vi "Main RT.vi"() -> ()   [LabVIEW 2015]
uses:
  <vilib>/RioEmbeddedCAN/RioEmbeddedCAN.llb/CANFrameControl.ctl
  <vilib>/Platform/TimedLoop/XDataNode/timing_clust.ctl
  <vilib>/Platform/TimedLoop/XDataNode/nitl_modes.ctl
  <vilib>/Platform/TimedLoop/XDataNode/wakeup.ctl
  <vilib>/FPGAPlugInAG/sbRIO-9636/niLvFpga_Open_sbRIO-9636.vi
  <vilib>/rvi/interface/common/dynamic/niFpgaDynamicAddResources.vi
  <vilib>/FPGAPlugInAG/Dynamic/niLvFpga_Reset_Dynamic.vi
  <vilib>/FPGAPlugInAG/Dynamic/niLvFpga_Run_Dynamic.vi
  <vilib>/FPGAPlugInAG/Dynamic/niLvFpga_Close_Dynamic.vi
  <vilib>/Platform/TimedLoop/XDataNode/XDataNode.xnode
  <vilib>/rvi/interface/nirviOpenFPGA/nirviOpenFPGA.xnode
  FPGA Bitfiles/Raptorv2_FPGATarget_FPGAMain_SQ-6zSZl0hY.lvbitx
  FPGA/Main FPGA.vi
  <vilib>/rvi/interface/nirviMethod/nirviMethod.xnode
  <vilib>/rvi/interface/nirviCloseFPGA/nirviCloseFPGA.xnode
  <vilib>/Platform/TimedLoop/XDataNode/XDNodeRunTimeDep.lvlib
  <vilib>/Instr/_visa.llb/VISA Configure Serial Port (Instr).vi
panel:
  out "longitude (deg) 2":dbl format="%#_8g"
  out "latitude (deg) 2":dbl format="%#_8g"
  in  "VISA resource name":refnum<visa-resource-name>="ASRL1::INSTR"
  out "longitude (deg)":i64
  out "latitude (deg)":i64
  out "GPS data":T1 {"oldest read timestamp" format="%^<%.3X\n%x>T"; "latitude (deg)" format="%#_10g"; "longitude (deg)" format="%#_10g"}
  out "Numeric 2":i32
  out "Numeric":i32
  out "okres 1000":dbl
  out "wyczyszczona":bool=TRUE
  in  "Wyczyśćkolejke":bool
  in  "stop wysylanie":bool
  out "odczytany CAN":T2 {"type" items=["CAN Data", "CAN Remote"]; "identifier" format="%.0x"}
  out "ile nowych mesagy":dbl
  in  "odczyt":bool=TRUE
  out "okres 100":dbl
  out "ilosc mesagy":dbl
  in  "ramki 2":bool
  out "Frames":string[][](table)
  in  "stop odczyt can":bool
  in  "Hexadecimal?":bool
  in  "stop zapis can":bool
  out "new data":bool
  out "ramki jazdy":T2[](array[typedef]) {"type" items=["CAN Data", "CAN Remote"]; "identifier" format="%.0x"}
  in  "odbior udp":bool
  out "ramki konf":T2 {"type" items=["CAN Data", "CAN Remote"]; "identifier" format="%.0x"}
  in  "Number of Frames to Display":i32=5
  in  "receive queue size":u32=500
  in  "baud rate":u32=500000
  in  "interface index":u32
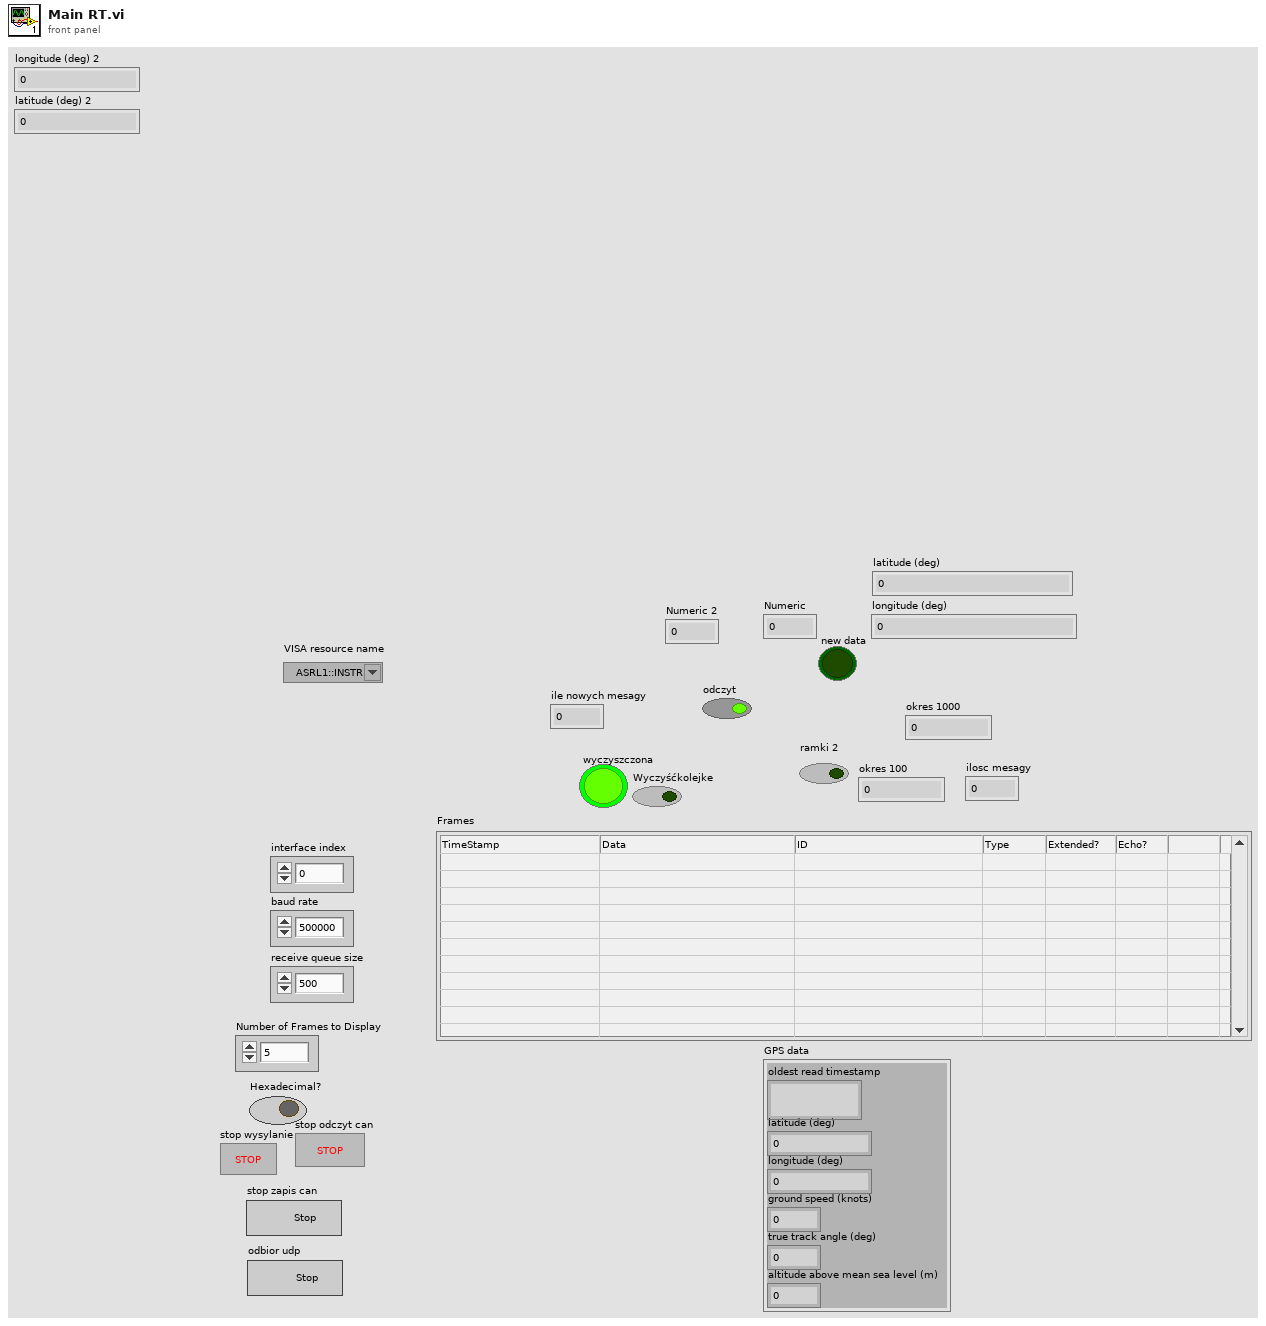
[diagram p1: front panel]
types:
  T1 = cluster{"oldest read timestamp":timestamp, "latitude (deg)":dbl, "longitude (deg)":dbl, "ground speed (knots)":dbl, "true track angle (deg)":dbl, "altitude above mean sea level (m)":dbl}
  T2 = typedef "CANFrameControl.ctl" = cluster{"identifier":u32, "extended?":bool, "type":u8, "payload":u8[]}
  T3 = typedef "XDNodeRunTimeDep.lvlib/timing_clust.ctl" = cluster{"Expected End [f-1]":u64, "Actual End [f-1]":u64, "Finished Late? [f-1]":bool, "Expected End [i-1]":u64, "Actual End [i-1]":u64, "Finished Late? [i-1]":bool, "Expected Start [i]":u64, "Actual Start [i]":u64, "Expected Start [f]":u64, "Actual Start [f]":u64, "Source Name":string, "Structure Name":string, "Period":i64, "Deadline":i64, "Offset":i64, "Start":i64, "Priority":i32, "Timeout":i32, "Mode":T4, "Wakeup Reason":T5, "Error":errorcluster, "Source Type":string, "Secondary Source Type":string, "Global End Time":u64, "Global Start Time":u64, "Frame Duration":u64, "Iteration Duration":u64, "Assigned CPU":i32, "I/O Scan Engine Mode":u32}
  T4 = typedef "XDNodeRunTimeDep.lvlib/nitl_modes.ctl" = enum32{"No Change", "Process missed periods, maintain original phase", "Discard missed periods, maintain original phase", "Process missed periods, ignore original phase", "Discard missed periods, ignore original phase"}
  T5 = typedef "XDNodeRunTimeDep.lvlib/wakeup.ctl" = enum32{"Normal", "Aborted", "Asynchronous wakeup", "Timing source error", "Timed loop error", "Timeout"}
  T6 = cluster{"latitude (deg)":i64, "longitude (deg)":i64}
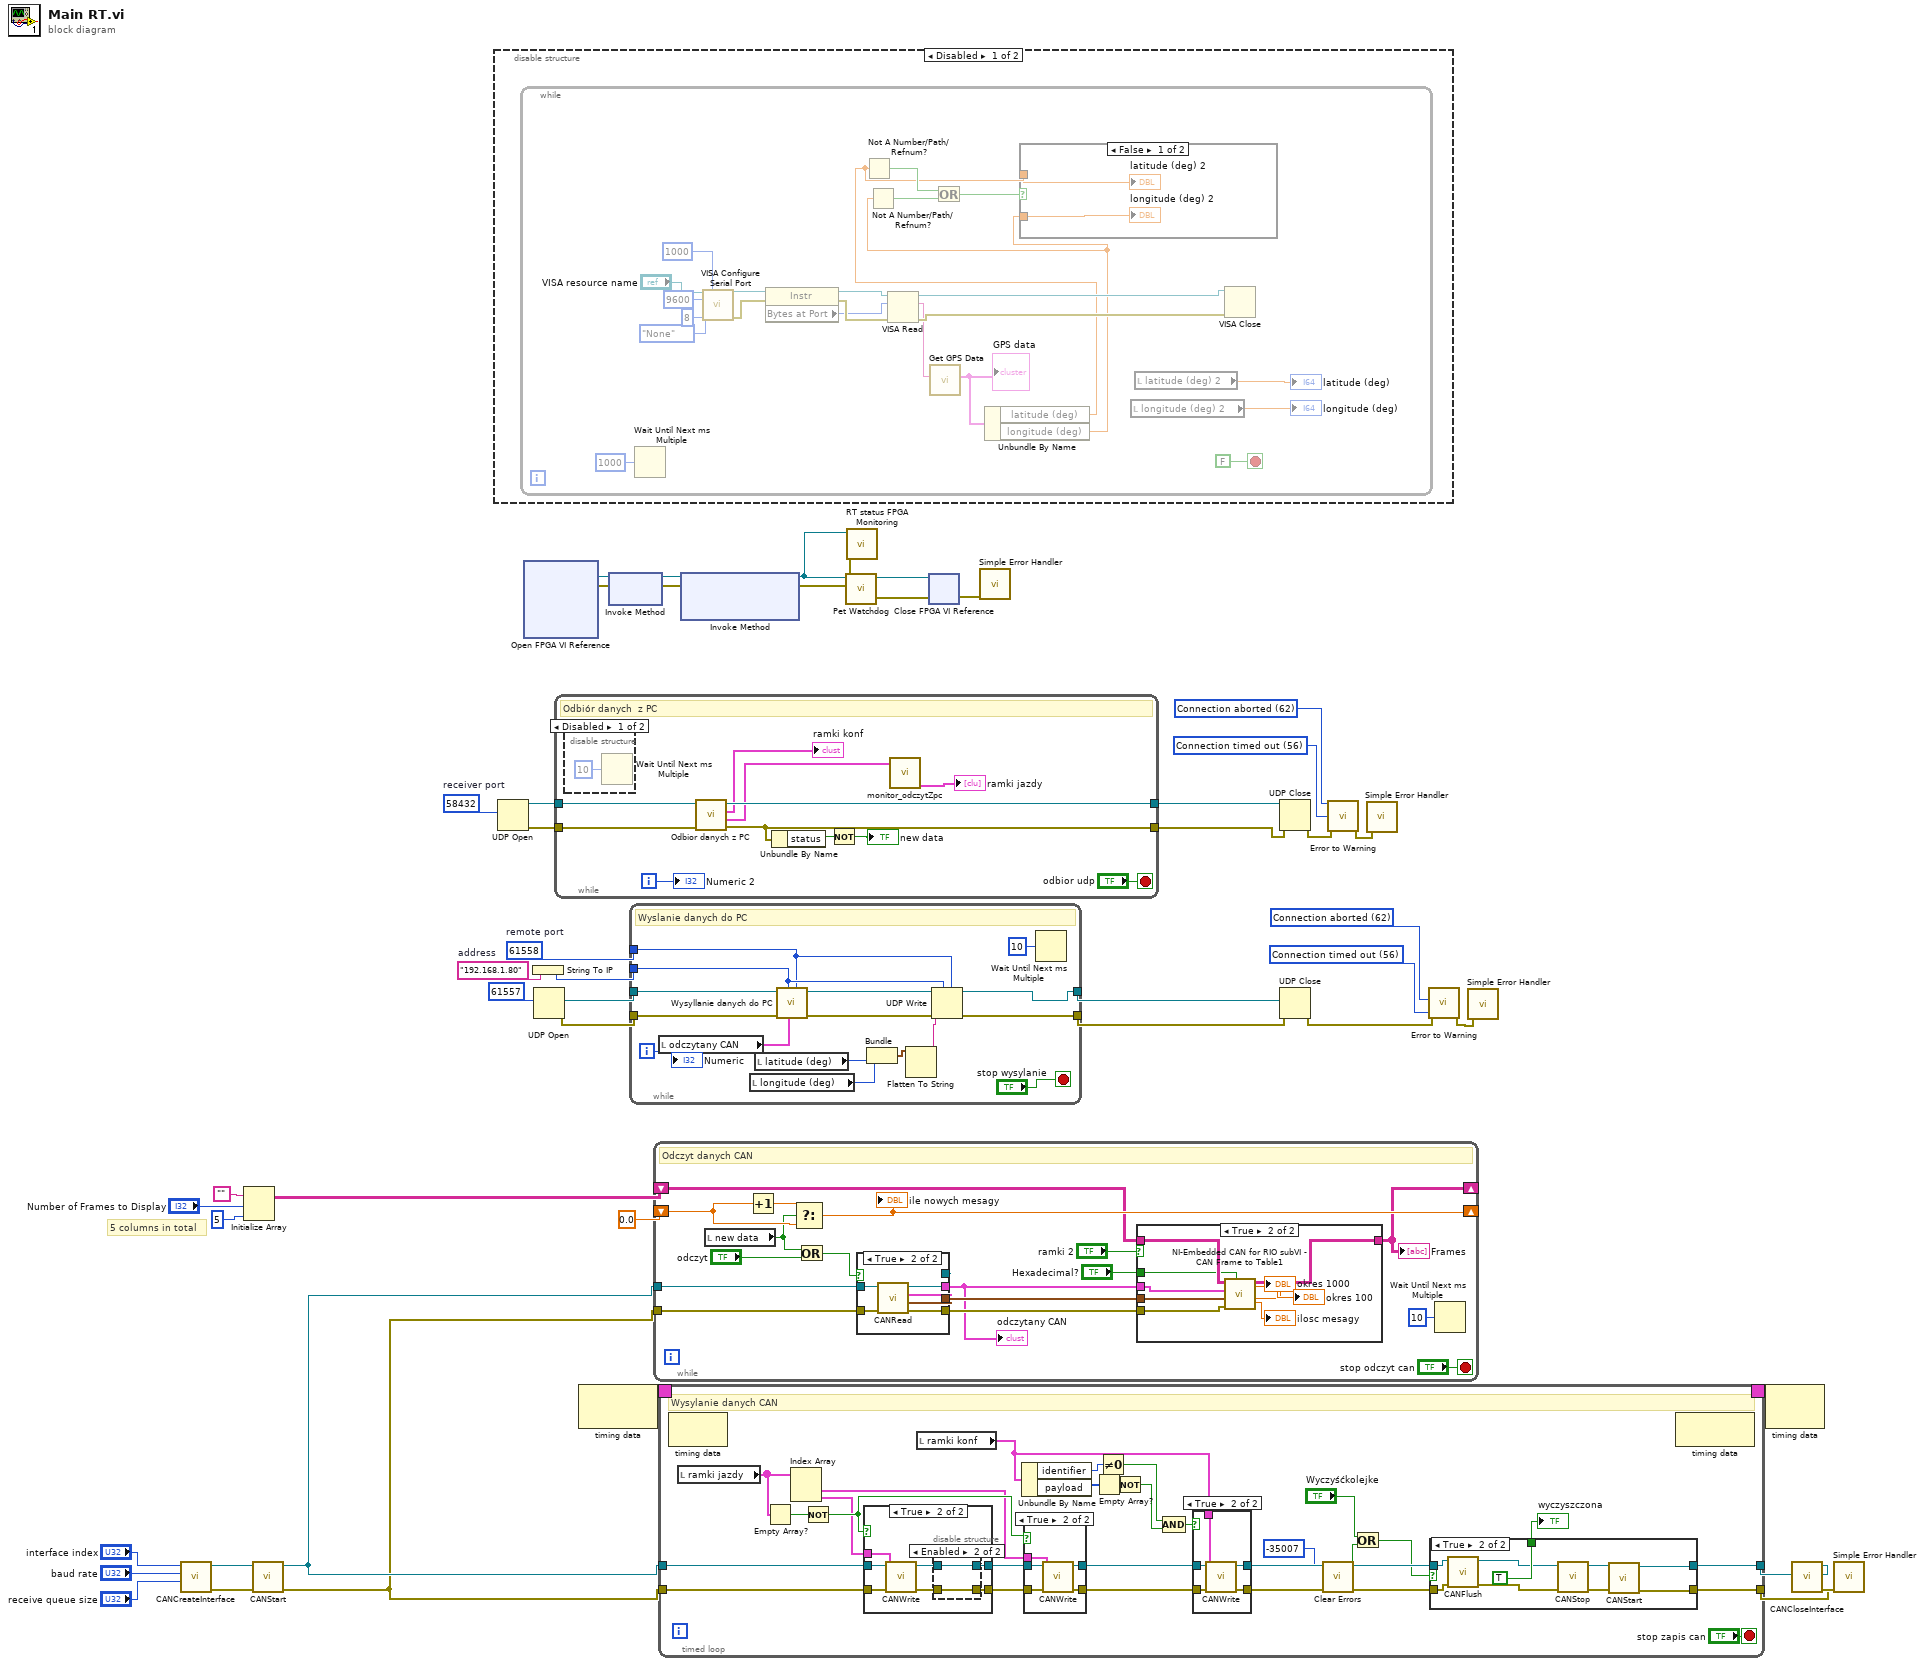
[diagram p0: block diagram]
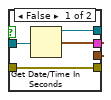
[diagram p6: hidden frame]
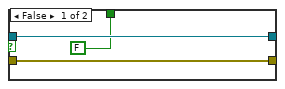
[diagram p7: hidden frame]
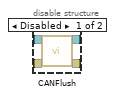
[diagram p11: hidden frame]
diagram:
  w2 = u16 58432  # receiver port
  w6 = 56 items=["No Error", "Argument Error", "Memory Full", "Out of Zone", "End of File", "File Already Open", "Generic File IO Error", "File Not Found", "File Permission Error", "Disk Full", "Duplicate Path", "Too Many Files Open", "Not Enabled", "Resource File Not Found", "Cannot Add Resource", "Resource Not Found", "Image Not Found", "Image Memory Error", "Pen Does Not Exist", "Config Bad Type", "Config Token Not Found", "Config Parse Error", "Config Memory Error", "Bad External Code Format", "Bad External Code Offset", "External Code Not Present", "Null Window", "Destroy Window Mixup", "Null Menu", "Print Aborted", "Bad Print Record", "Print Driver Error", "Windows Error During Print", "Memory Error During Print", "Print Dialog Error", "Generic Print Error", "Invalid Device Refnum", "Device Not Found", "Device Parameter Error", "Device Unit Error", "Can't Open Device", "Device Call Aborted", "Generic Error", "Cancelled By User", "Object ID Too Low", "Object ID Too High", "Object Not In Heap", "Unknown Heap", "Bad DefProc ID", "DefProc Not In Table", "Message Out Of Range", "Null Method", "Unknown Message", "Manager Call Not Supported", "Bad address", "Connection In progress", "Connection timed out", "Connection is already in progress", "Network attribute not supported", "Network error", "Address in use", "System out of memory", "Connection aborted", "Connection refused", "Connection is not connected", "Connection is already connected", "Connection closed", "Initialize error (interapplication manager)", "Bad occurrence", "Wait on unbound occurrence handler", "Occurrence queue overflow", "Bad path", "Semaphore not signaled", "Unrecognized type (interapplication manager)"] ("3rd Error to Convert")
  w5 = 62 items=["No Error", "Argument Error", "Memory Full", "Out of Zone", "End of File", "File Already Open", "Generic File IO Error", "File Not Found", "File Permission Error", "Disk Full", "Duplicate Path", "Too Many Files Open", "Not Enabled", "Resource File Not Found", "Cannot Add Resource", "Resource Not Found", "Image Not Found", "Image Memory Error", "Pen Does Not Exist", "Config Bad Type", "Config Token Not Found", "Config Parse Error", "Config Memory Error", "Bad External Code Format", "Bad External Code Offset", "External Code Not Present", "Null Window", "Destroy Window Mixup", "Null Menu", "Print Aborted", "Bad Print Record", "Print Driver Error", "Windows Error During Print", "Memory Error During Print", "Print Dialog Error", "Generic Print Error", "Invalid Device Refnum", "Device Not Found", "Device Parameter Error", "Device Unit Error", "Can't Open Device", "Device Call Aborted", "Generic Error", "Cancelled By User", "Object ID Too Low", "Object ID Too High", "Object Not In Heap", "Unknown Heap", "Bad DefProc ID", "DefProc Not In Table", "Message Out Of Range", "Null Method", "Unknown Message", "Manager Call Not Supported", "Bad address", "Connection In progress", "Connection timed out", "Connection is already in progress", "Network attribute not supported", "Network error", "Address in use", "System out of memory", "Connection aborted", "Connection refused", "Connection is not connected", "Connection is already connected", "Connection closed", "Initialize error (interapplication manager)", "Bad occurrence", "Wait on unbound occurrence handler", "Occurrence queue overflow", "Bad path", "Semaphore not signaled", "Unrecognized type (interapplication manager)"] ("1st Error to Convert")
  w13 = u16 61558  # remote port
  w14 = "192.168.1.80"  # address
  w17 = 56 items=["No Error", "Argument Error", "Memory Full", "Out of Zone", "End of File", "File Already Open", "Generic File IO Error", "File Not Found", "File Permission Error", "Disk Full", "Duplicate Path", "Too Many Files Open", "Not Enabled", "Resource File Not Found", "Cannot Add Resource", "Resource Not Found", "Image Not Found", "Image Memory Error", "Pen Does Not Exist", "Config Bad Type", "Config Token Not Found", "Config Parse Error", "Config Memory Error", "Bad External Code Format", "Bad External Code Offset", "External Code Not Present", "Null Window", "Destroy Window Mixup", "Null Menu", "Print Aborted", "Bad Print Record", "Print Driver Error", "Windows Error During Print", "Memory Error During Print", "Print Dialog Error", "Generic Print Error", "Invalid Device Refnum", "Device Not Found", "Device Parameter Error", "Device Unit Error", "Can't Open Device", "Device Call Aborted", "Generic Error", "Cancelled By User", "Object ID Too Low", "Object ID Too High", "Object Not In Heap", "Unknown Heap", "Bad DefProc ID", "DefProc Not In Table", "Message Out Of Range", "Null Method", "Unknown Message", "Manager Call Not Supported", "Bad address", "Connection In progress", "Connection timed out", "Connection is already in progress", "Network attribute not supported", "Network error", "Address in use", "System out of memory", "Connection aborted", "Connection refused", "Connection is not connected", "Connection is already connected", "Connection closed", "Initialize error (interapplication manager)", "Bad occurrence", "Wait on unbound occurrence handler", "Occurrence queue overflow", "Bad path", "Semaphore not signaled", "Unrecognized type (interapplication manager)"] ("3rd Error to Convert")
  w18 = 62 items=["No Error", "Argument Error", "Memory Full", "Out of Zone", "End of File", "File Already Open", "Generic File IO Error", "File Not Found", "File Permission Error", "Disk Full", "Duplicate Path", "Too Many Files Open", "Not Enabled", "Resource File Not Found", "Cannot Add Resource", "Resource Not Found", "Image Not Found", "Image Memory Error", "Pen Does Not Exist", "Config Bad Type", "Config Token Not Found", "Config Parse Error", "Config Memory Error", "Bad External Code Format", "Bad External Code Offset", "External Code Not Present", "Null Window", "Destroy Window Mixup", "Null Menu", "Print Aborted", "Bad Print Record", "Print Driver Error", "Windows Error During Print", "Memory Error During Print", "Print Dialog Error", "Generic Print Error", "Invalid Device Refnum", "Device Not Found", "Device Parameter Error", "Device Unit Error", "Can't Open Device", "Device Call Aborted", "Generic Error", "Cancelled By User", "Object ID Too Low", "Object ID Too High", "Object Not In Heap", "Unknown Heap", "Bad DefProc ID", "DefProc Not In Table", "Message Out Of Range", "Null Method", "Unknown Message", "Manager Call Not Supported", "Bad address", "Connection In progress", "Connection timed out", "Connection is already in progress", "Network attribute not supported", "Network error", "Address in use", "System out of memory", "Connection aborted", "Connection refused", "Connection is not connected", "Connection is already connected", "Connection closed", "Initialize error (interapplication manager)", "Bad occurrence", "Wait on unbound occurrence handler", "Occurrence queue overflow", "Bad path", "Semaphore not signaled", "Unrecognized type (interapplication manager)"] ("1st Error to Convert")
  # "5 columns in total"
  n1 = call <vilib>:"CANCreateInterface.vi"("receive queue size (5)"="receive queue size", "baud rate (125000 bps)"="baud rate", "interface index"="interface index") -> ("error out"=w45:errorcluster, "interface object out"=w35:refnum<k20>)  [unwired: 7 in]
  n2 = Initialize Array("" ("Empty String Constant"), "Number of Frames to Display", 5 ("dimension size")) -> (w34:string[][])
  n3 = call <vilib>:"CANStart.vi"("error in (no error)"=w45, "interface object in"=w35) -> ("error out"=w32:errorcluster, "interface object out"=w33:refnum<k20>)  [unwired: 8 in]
  n4 = disable-structure shown="Disabled" {
    frame Disabled {
      n5 = while {
        stop <- FALSE stop-if-true
        n6 = Wait Until Next ms Multiple(millisecond multiple=u32 1000) -> ()  [unwired: 1 out]
        n7 = call-poly "VISA Configure Serial Port"("VISA resource name"="VISA resource name", "timeout (10sec)"=u32 1000, "baud rate (9600)"=u32 9600, "data bits (8)"=u16 8, "parity (0:none)"=enum16{"None", "Odd", "Even", "Mark", "Space"}."None") -> ("VISA resource name out"=w67:refnum<visa-resource-name>, "error out"=w66:errorcluster)  [unwired: 9 in]
        n8 = property class="Instr"(reference=w67, error in=w66) -> (reference out=w68:refnum<visa-resource-name>, error out=w65:errorcluster, "Bytes at Port"=w61:u32)
        n9 = VISA Read(VISA resource name=w68, byte count=w61, error in (no error)=w65) -> (VISA resource name out=w69:refnum<visa-resource-name>, read buffer=w63:string, error out=w64:errorcluster)  [unwired: 1 out]
        n10 = call <vilib>:"Get GPS Data.vi"("sensor data"=w63) -> ("GPS data"=w62:T1)  [unwired: 8 in, 2 out]
        "GPS data" <- w62
        n11 = Unbundle By Name(w62) -> ("latitude (deg)"=w51:dbl, "longitude (deg)"=w49:dbl)
        n12 = Not A Number/Path/Refnum?(number/path/refnum=w51) -> (NaN/Path/Refnum?=w54:bool)
        n13 = Not A Number/Path/Refnum?(number/path/refnum=w49) -> (NaN/Path/Refnum?=w53:bool)
        n14 = Or(x=w54, y=w53) -> (x .or. y?=w52:bool)
        n15 = case shown="False" w52 {
          tunnel: w49 -> [w72 _]
          tunnel: w51 -> [w71 _]
          frame False {
            "longitude (deg) 2" <- w72
            "latitude (deg) 2" <- w71
          }
          frame True {
          }
        }
        n16 = local read "longitude (deg) 2"() -> (→"longitude (deg)":dbl)
        n17 = local read "latitude (deg) 2"() -> (→"latitude (deg)":dbl)
        n18 = VISA Close(VISA resource name=w69, error in (no error)=w64) -> ()  [unwired: 1 out]
      }
    }
    frame Enabled {
    }
  }
  n19 = UDP Open(11:w2) -> (port=w20:refnum<k16>, 0:w21:errorcluster)  [unwired: 4 in, 1 out]
  n20 = xnode "Open FPGA VI Reference"() -> ("FPGA VI Reference Out"=w26:refnum<k20>, "error out"=w27:errorcluster)  [unwired: 2 in]
  n21 = String To IP(1:w14) -> (0:w12:u32)
  n22 = UDP Open(11:u16 61557 ("port")) -> (port=w11:refnum<k16>, 0:w10:errorcluster)  [unwired: 4 in, 1 out]
  n23 = while {
    tunnel: w20 -> [w80]
    tunnel: w21 -> [w79]
    tunnel: [w82] -> w22
    tunnel: [w83] -> w3
    i -> [w78]
    stop <- "odbior udp" stop-if-true
    # "Odbiór danych  z PC"
    n24 = disable-structure shown="Disabled" {
      frame Disabled {
        n25 = Wait Until Next ms Multiple(millisecond multiple=u32 10) -> ()  [unwired: 1 out]
      }
      frame Enabled {
      }
    }
    n26 = call "Odbior danych z PC .vi"("error in (no error)"=w79, "connection ID"=w80) -> ("error out"=w82:errorcluster, "jazda"=w75:T2[], "konf"=→"ramki konf":T2, "connection ID out"=w83:refnum<k16>)  [unwired: 6 in]
    n27 = Unbundle By Name(w82) -> ("status"=w77:bool)
    n28 = Not(x=w77) -> (.not. x?=→"new data":bool)
    n29 = call "monitor_odczytZpc.vi"("ramki jazdy 2"=w75) -> ("ramki jazdy out"=→"ramki jazdy":T2[])  [unwired: 9 in, 1 out]
    "Numeric 2" <- w78
  }
  n30 = node-c288() -> (w47:T3)  [unwired: 1 in]
  n31 = xnode "Invoke Method"("FPGA VI Reference In"=w26, "error in"=w27) -> ("FPGA VI Reference Out"=w28:refnum<k20>, "error out"=w29:errorcluster)
  n32 = while {
    tunnel: w13 -> [w87]
    tunnel: w12 -> [w88]
    tunnel: w11 -> [w100]
    tunnel: w10 -> [w99]
    tunnel: [w86] -> w9
    tunnel: [w85] -> w8
    i -> [w95]
    stop <- "stop wysylanie" stop-if-true
    # "Wyslanie danych do PC"
    n33 = local read "odczytany CAN"() -> (w96:T2)
    n34 = local read "longitude (deg)"() -> (w89:i64)
    n35 = local read "latitude (deg)"() -> (w90:i64)
    n36 = call "Wysyllanie danych do PC .vi"("remote port"=w87, "odczytany CAN"=w96, "Numeric"=w88, "error in (no error)"=w99, "UDP Network Connection in"=w100) -> ("error out"=w94:errorcluster, "UDP Network Connection out"=w93:refnum<k16>)  [unwired: 5 in]
    n37 = Bundle("latitude (deg)"=w90, "longitude (deg)"=w89) -> (w91:T6)  [unwired: 1 in]
    n38 = Flatten To String(anything=w91) -> (data string=w92:string)  [unwired: 3 in, 2 out]
    n39 = UDP Write(address=w88, port or service name=w87, connection ID=w93, data in=w92, 8:w94) -> (error out=w85:errorcluster, 3:w86:refnum<k16>)  [unwired: 1 in]
    n40 = Wait Until Next ms Multiple(millisecond multiple=u32 10) -> ()  [unwired: 1 out]
    "Numeric" <- w95
  }
  n41 = while {
    shift-right: [w109] -> _
    shift-left: w34 -> [w108]
    shift-right: [w113] -> _
    shift-left: 0.0 -> [w114]
    tunnel: w33 -> [w117]
    tunnel: w32 -> [w116]
    stop <- "stop odczyt can" stop-if-true
    # "Odczyt danych CAN"
    n42 = local read "new data"() -> (w111:bool)
    n43 = Increment(x=w114) -> (x+1=w115:dbl)
    n44 = Select(t=w115, s=w111, f=w114) -> (s? t:f=w113:dbl)
    "ile nowych mesagy" <- w113
    n45 = Or(x=w111, y="odczyt") -> (x .or. y?=w110:bool)
    n46 = case shown="True" w110 {
      tunnel: w117 -> [w129 w136]
      tunnel: w116 -> [w130 w135]
      tunnel: [w128 w134] -> w107
      tunnel: [w130 w133] -> w106
      tunnel: [_ w131] -> w101
      tunnel: [w129 w132] -> _
      frame False {
        n47 = Get Date/Time In Seconds() -> (seconds since 1Jan1904=w128:timestamp)
      }
      frame True {
        n48 = call <vilib>:"CANRead.vi"("error in (no error)"=w135, "interface object in"=w136) -> ("error out"=w133:errorcluster, "timestamp"=w134:timestamp, "CAN frame"=w131:T2, "interface object out"=w132:refnum<k20>)  [unwired: 6 in]
      }
    }
    "odczytany CAN" <- w101
    n49 = case shown="True" "ramki 2" {
      tunnel: [w118 w127] -> w109
      tunnel: w108 -> [w118 w124]
      tunnel: w107 -> [_ w123]
      tunnel: w101 -> [_ w122]
      tunnel: w106 -> [_ w121]
      tunnel: "Hexadecimal?" -> [_ w120]
      frame False {
      }
      frame True {
        n50 = call "NI-Embedded CAN for RIO subVI - CAN Frame to Table1.vi"("Hexadecimal?"=w120, "error in (no error)"=w121, "timestamp"=w123, "CAN frame"=w122, "Input Array"=w124) -> ("okres 1000"=→"okres 1000":dbl, "Output Array"=w127:string[][], "ilosc mesagy"=→"ilosc mesagy":dbl, "okres 100"=→"okres 100":dbl)  [unwired: 2 in, 1 out]
      }
    }
    "Frames" <- w109
    n51 = Wait Until Next ms Multiple(millisecond multiple=u32 10) -> ()  [unwired: 1 out]
  }
  n52 = timed-loop "Timed Loop" {
    tunnel: w33 -> [w148]
    tunnel: w32 -> [w147]
    tunnel: [w146] -> w37
    tunnel: [w145] -> w36
    timing: w47 -> [_]
    timing-out: [_] -> w46
    stop <- "stop zapis can" stop-if-true
    # "Wysylanie danych CAN"
    n53 = node-c288() -> ()  [unwired: 1 in, 1 out]
    n54 = local read "ramki jazdy"() -> (w163:T2[])
    n55 = Empty Array?(array=w163) -> (empty?=w162:bool)
    n56 = Index Array(array=w163) -> (element #1=w160:T2, element #2=w159:T2)  [unwired: 2 in]
    n57 = Not(x=w162) -> (.not. x?=w161:bool)
    n58 = case shown="True" w161 {
      tunnel: w148 -> [w194 w202]
      tunnel: w147 -> [w195 w201]
      tunnel: [w194 w196] -> w164
      tunnel: [w195 w197] -> w165
      tunnel: w159 -> [_ w200]
      frame False {
      }
      frame True {
        n59 = call <vilib>:"CANWrite.vi"("error in (no error)"=w201, "CAN frame"=w200, "interface object in"=w202) -> ("error out"=w199:errorcluster, "interface object out"=w198:refnum<k20>)  [unwired: 7 in]
        n60 = disable-structure shown="Enabled" {
          disable-tunnel: w199 -> [w206 w207]
          disable-tunnel: w198 -> [w205 w208]
          disable-tunnel: [w204 w207] -> w197
          disable-tunnel: [w203 w208] -> w196
          frame Disabled {
            n61 = call <vilib>:"CANFlush.vi"("error in (no error)"=w206, "interface object in"=w205) -> ("error out"=w204:errorcluster, "interface object out"=w203:refnum<k20>)  [unwired: 8 in]
          }
          frame Enabled {
          }
        }
      }
    }
    n62 = local read "ramki konf"() -> (w156:T2)
    n63 = Unbundle By Name(w156) -> ("identifier"=w154:u32, "payload"=w155:u8[])
    n64 = case shown="True" w161 {
      tunnel: w165 -> [w188 w193]
      tunnel: [w187 w190] -> w158
      tunnel: [w188 w189] -> w157
      tunnel: w164 -> [w187 w192]
      tunnel: w160 -> [_ w191]
      frame False {
      }
      frame True {
        n65 = call <vilib>:"CANWrite.vi"("error in (no error)"=w193, "CAN frame"=w191, "interface object in"=w192) -> ("error out"=w189:errorcluster, "interface object out"=w190:refnum<k20>)  [unwired: 7 in]
      }
    }
    n66 = Empty Array?(array=w155) -> (empty?=w151:bool)
    n67 = Not Equal To 0?(x=w154) -> (x != 0?=w152:bool)
    n68 = Not(x=w151) -> (.not. x?=w150:bool)
    n69 = Compound Arithmetic op=AND(w152, w150) -> (w153:bool)
    n70 = case shown="True" w153 {
      tunnel: w157 -> [w179 w184]
      tunnel: [w178 w181] -> w144
      tunnel: [w179 w180] -> w149
      tunnel: w158 -> [w178 w183]
      tunnel: w156 -> [_ w182]
      frame False {
      }
      frame True {
        n71 = call <vilib>:"CANWrite.vi"("error in (no error)"=w184, "CAN frame"=w182, "interface object in"=w183) -> ("error out"=w180:errorcluster, "interface object out"=w181:refnum<k20>)  [unwired: 7 in]
      }
    }
    n72 = call <vilib>:"Clear Errors.vi"("error in (no error)"=w149, "specific error code to clear (0: all)"=-35007) -> ("error out"=w141:errorcluster, "specific error cleared?"=w139:bool)  [unwired: 4 in]
    n73 = Or(x="Wyczyśćkolejke", y=w139) -> (x .or. y?=w140:bool)
    n74 = case shown="True" w140 {
      tunnel: [w168 w170] -> w146
      tunnel: [w167 w169] -> w145
      tunnel: w144 -> [w168 w177]
      tunnel: w141 -> [w167 w176]
      tunnel: [FALSE TRUE] -> w137
      frame False {
      }
      frame True {
        n75 = call <vilib>:"CANFlush.vi"("error in (no error)"=w176, "interface object in"=w177) -> ("error out"=w173:errorcluster, "interface object out"=w174:refnum<k20>)  [unwired: 8 in]
        n76 = call <vilib>:"CANStop.vi"("error in (no error)"=w173, "interface object in"=w174) -> ("error out"=w172:errorcluster, "interface object out"=w171:refnum<k20>)  [unwired: 8 in]
        n77 = call <vilib>:"CANStart.vi"("error in (no error)"=w172, "interface object in"=w171) -> ("error out"=w169:errorcluster, "interface object out"=w170:refnum<k20>)  [unwired: 8 in]
      }
    }
    "wyczyszczona" <- w137
    n78 = node-c288() -> ()  [unwired: 1 in, 1 out]
  }
  n79 = xnode "Invoke Method"("FPGA VI Reference In"=w28, "error in"=w29) -> ("FPGA VI Reference Out"=w1:refnum<k20>, "error out"=w24:errorcluster)  [unwired: 1 in]
  n80 = call "Pet Watchdog.vi"("error in (no error)"=w24, "FPGA VI Reference Out"=w1) -> ("error out"=w30:errorcluster, "FPGA VI Reference Out 2"=w23:refnum<k20>)  [unwired: 8 in]
  n81 = call "RT status FPGA Monitoring.vi"("error in (no error)"=w24, "FPGA VI Reference Out 2"=w1) -> ()  [unwired: 10 in]
  n82 = xnode "Close FPGA VI Reference"("FPGA VI Reference In"=w23, "error in"=w30) -> ("error out"=w25:errorcluster)
  n83 = call <vilib>:"Simple Error Handler.vi"("error in (no error)"=w25) -> ()  [unwired: 1 in, 8 out]
  n84 = UDP Close(connection ID=w3, 8:w22) -> (error out=w4:errorcluster)  [unwired: 1 out]
  n85 = UDP Close(connection ID=w9, 8:w8) -> (error out=w19:errorcluster)  [unwired: 1 out]
  n86 = call <vilib>:"Error to Warning.vi"("1st Error to Convert"=w5, "3rd Error to Convert"=w6, "error in"=w4) -> ("warning out"=w7:errorcluster)  [unwired: 3 in, 9 out]
  n87 = call <vilib>:"Simple Error Handler.vi"("error in (no error)"=w7) -> ()  [unwired: 1 in, 8 out]
  n88 = call <vilib>:"Error to Warning.vi"("1st Error to Convert"=w18, "3rd Error to Convert"=w17, "error in"=w19) -> ("warning out"=w16:errorcluster)  [unwired: 3 in, 9 out]
  n89 = call <vilib>:"Simple Error Handler.vi"("error in (no error)"=w16) -> ()  [unwired: 1 in, 8 out]
  n90 = node-c288(w46) -> ()  [unwired: 1 out]
  n91 = call <vilib>:"CANCloseInterface.vi"("error in (no error)"=w36, "interface object in"=w37) -> ("error out"=w38:errorcluster)  [unwired: 9 in]
  n92 = call <vilib>:"Simple Error Handler.vi"("error in (no error)"=w38) -> ()  [unwired: 4 in, 5 out]
